vi "nanocal -- nuclear schottky fit V3.vi"() -> ()   [LabVIEW 2020] (continued)
  T4 = typedef "nameformattingitem.ctl" = enum16{"name", "nameL", "units", "prec"}
  T5 = typedef "nanocal-goodness-weighting-strategy.ctl" = enum16{"dω", "dω √(|dz/dω|)", "dω |dz/dω|", "phase", "andreas", "sum"}
  T6 = typedef "3-lorentzian-heat-response action.ctl" = enum16{"calc R", "create string", "calc m1m2m3", "dζ", "dT1", "dτS", "dτN", "dτC", "d-all", "dκ0", "T(K)", "m1", "m2", "m3", "parse string", "θ (deg)", "B (T)", "onlygrads", "newton", "create emty string"}
  T7 = enum32{"main", "parameters", "ignore", "save scan"}
  T8 = typedef "cursor winow.ctl" = cluster{"left":dbl, "right ":dbl, "center":dbl, "window":dbl, "cursors":i32[], "relative":i32, "absolute":i32, "fixed vertical offset":dbl, "vertical offset":dbl, "skew":dbl, "default window frac":dbl, "kind":enum16{"symmetric", "skewed", "fancy"}, "skew.left":dbl, "skew.right":dbl, "Plot ref":refnum<vi>, "wing order":enum16{"forw", "back"}}
  T9 = typedef "show-win- control.ctl" = cluster{"cen (Hz)":dbl, "win (Hz)":dbl, "left (Hz)":dbl, "right (Hz)":dbl}
  T10 = typedef "NI_Gmath.lvlib/stopping criteria.ctl" = cluster{"function tolerance":dbl, "parameter tolerance":dbl, "max iterations":i32, "max function calls":i32, "gradient tolerance":dbl, "max time (sec)":dbl}
  T11 = typedef "filename-pattern.ctl" = cluster{"prefix":string, "group":string}
  T12 = typedef "cursor action.ctl" = enum16{"range", "read", "write", "check", "zoom out", "smart zoom out", "zoom to aspect ratio 1", "zoom to win", "zoom out 20%", "zoom in 20%", "-empty", "smart zoom out&aspect", "move range left 20%", "move range right 20%", "move range up 20%", "move range down 20%", "zoom to X win", "zoom to Y win", "zoom out X", "zoom out Y", "zoom in X", "zoom in Y", "check plot scale", "set color", "set Xlabel", "set Ylabel"}
  T13 = typedef "cursor window action.ctl" = enum16{"balance", "h. offset change", "cursor moves", "change center", "change window", "init", "check", "reset", "set y to middle", "idle", "-write all Y", "-write left.X", "-write center.X", "-write right.X", "-write all X", "-change center", "-change window", "-change skew", "-read cursor 2", "-read cursor 1", "-read cursor 0", "-read all cursors", "-reset", "-read plot scale", "-set y to middle", "-Q: center.Y is visible", "-Q: window is visible", "-parse center.Y", "-right left from center", "-left move", "-right move", "-set center.Y", "-empty", "-set cursors to default", "-check", "-write center.Y", "-copy cursor 1", "-copy cursor 0", "-copy cursor 2", "move right", "move left", "shrink", "broaden", "skew up", "skew down", "-write plot scale", "zoom X", "change cen&win", "zoom to all data", "color--red", "color--green", "color--yellow", "read", "zoom out", "zoom in", "slide right", "slide left", "set range aspect ratio to 1"}
  T14 = typedef "mathematica string map action.ctl" = enum16{"create string", "calc m1m2m3", "parse string"}
  T15 = typedef "publisher action.ctl" = enum16{"set", "get", "init", "check"}
  T16 = typedef "cursor sate.ctl" = enum16{"normal", "alert", "fuzzy", "interesting", "boring", "colored"}
  T17 = typedef "3-lorentzian-parameters -- action.ctl" = enum16{"to array", "to parameters"}
  T18 = typedef "NI_Gmath.lvlib/objective function data.ctl" = variant
  T19 = typedef "filename-action.ctl" = enum16{"rewrite", "parse", "force pattern", "uniquenum", "get T", "get B", "get ind", "get deg", "get name", "get folder", "get extension", "get basename", "get side", "get change"}
  T20 = typedef "LVMapReplaceAction.ctl" = enum32{"Modify Entry only if found", "Add or Modify Entry", "Delete Entry"}
  T21 = typedef "file -- read-write control.ctl" = enum16{"read", "write all", "append one line"}
  T22 = typedef "array -- freq-voltage transformations action.ctl" = enum16{"as is", "add -ω", "sort ω", "2 x ω", "R-phase(deg) to Re-Im", "select ω>0"}
  T23 = typedef "nanocal_raw_file_manage_action_V1.ctl" = enum16{"read S side", "read R side", "read meta", "read_names"}
  T24 = typedef "KM_file -- read-write control.ctl" = enum16{"read", "write all", "append one line"}
  T25 = typedef "array action.ctl" = enum16{"generate range", "generate log range"}
  T26 = typedef "LVRangeTypeDef.ctl" = cluster{"Minimum":dbl, "Maximum":dbl, "Increment":dbl, "Minor Increment":dbl, "Start":dbl}
  T27 = typedef "2Dwindow.ctl" = cluster{"window y":dbl, "center x":dbl, "center y":dbl, "window x":dbl}
  T28 = typedef "eventvkey.ctl" = enum16{"ASCII", "Enter", "Return", "Shift", "Ctrl", "Alt", "Cmd", "Opt", "Caps", "NumLock", "Clear", "Break", "Up", "Down", "Left", "Right", "Insert", "Delete", "Home", "End", "PageUp", "PageDown", "Escape", "Help", "Pause", "ScrollLock", "F1", "F2", "F3", "F4", "F5", "F6", "F7", "F8", "F9", "F10", "F11", "F12", "F13", "F14", "F15", "F16", "F17", "F18", "F19", "F20", "F21", "F22", "F23", "F24", "Play", "VolumeUp", "VolumeDown", "Mute", "Two Byte Char"}
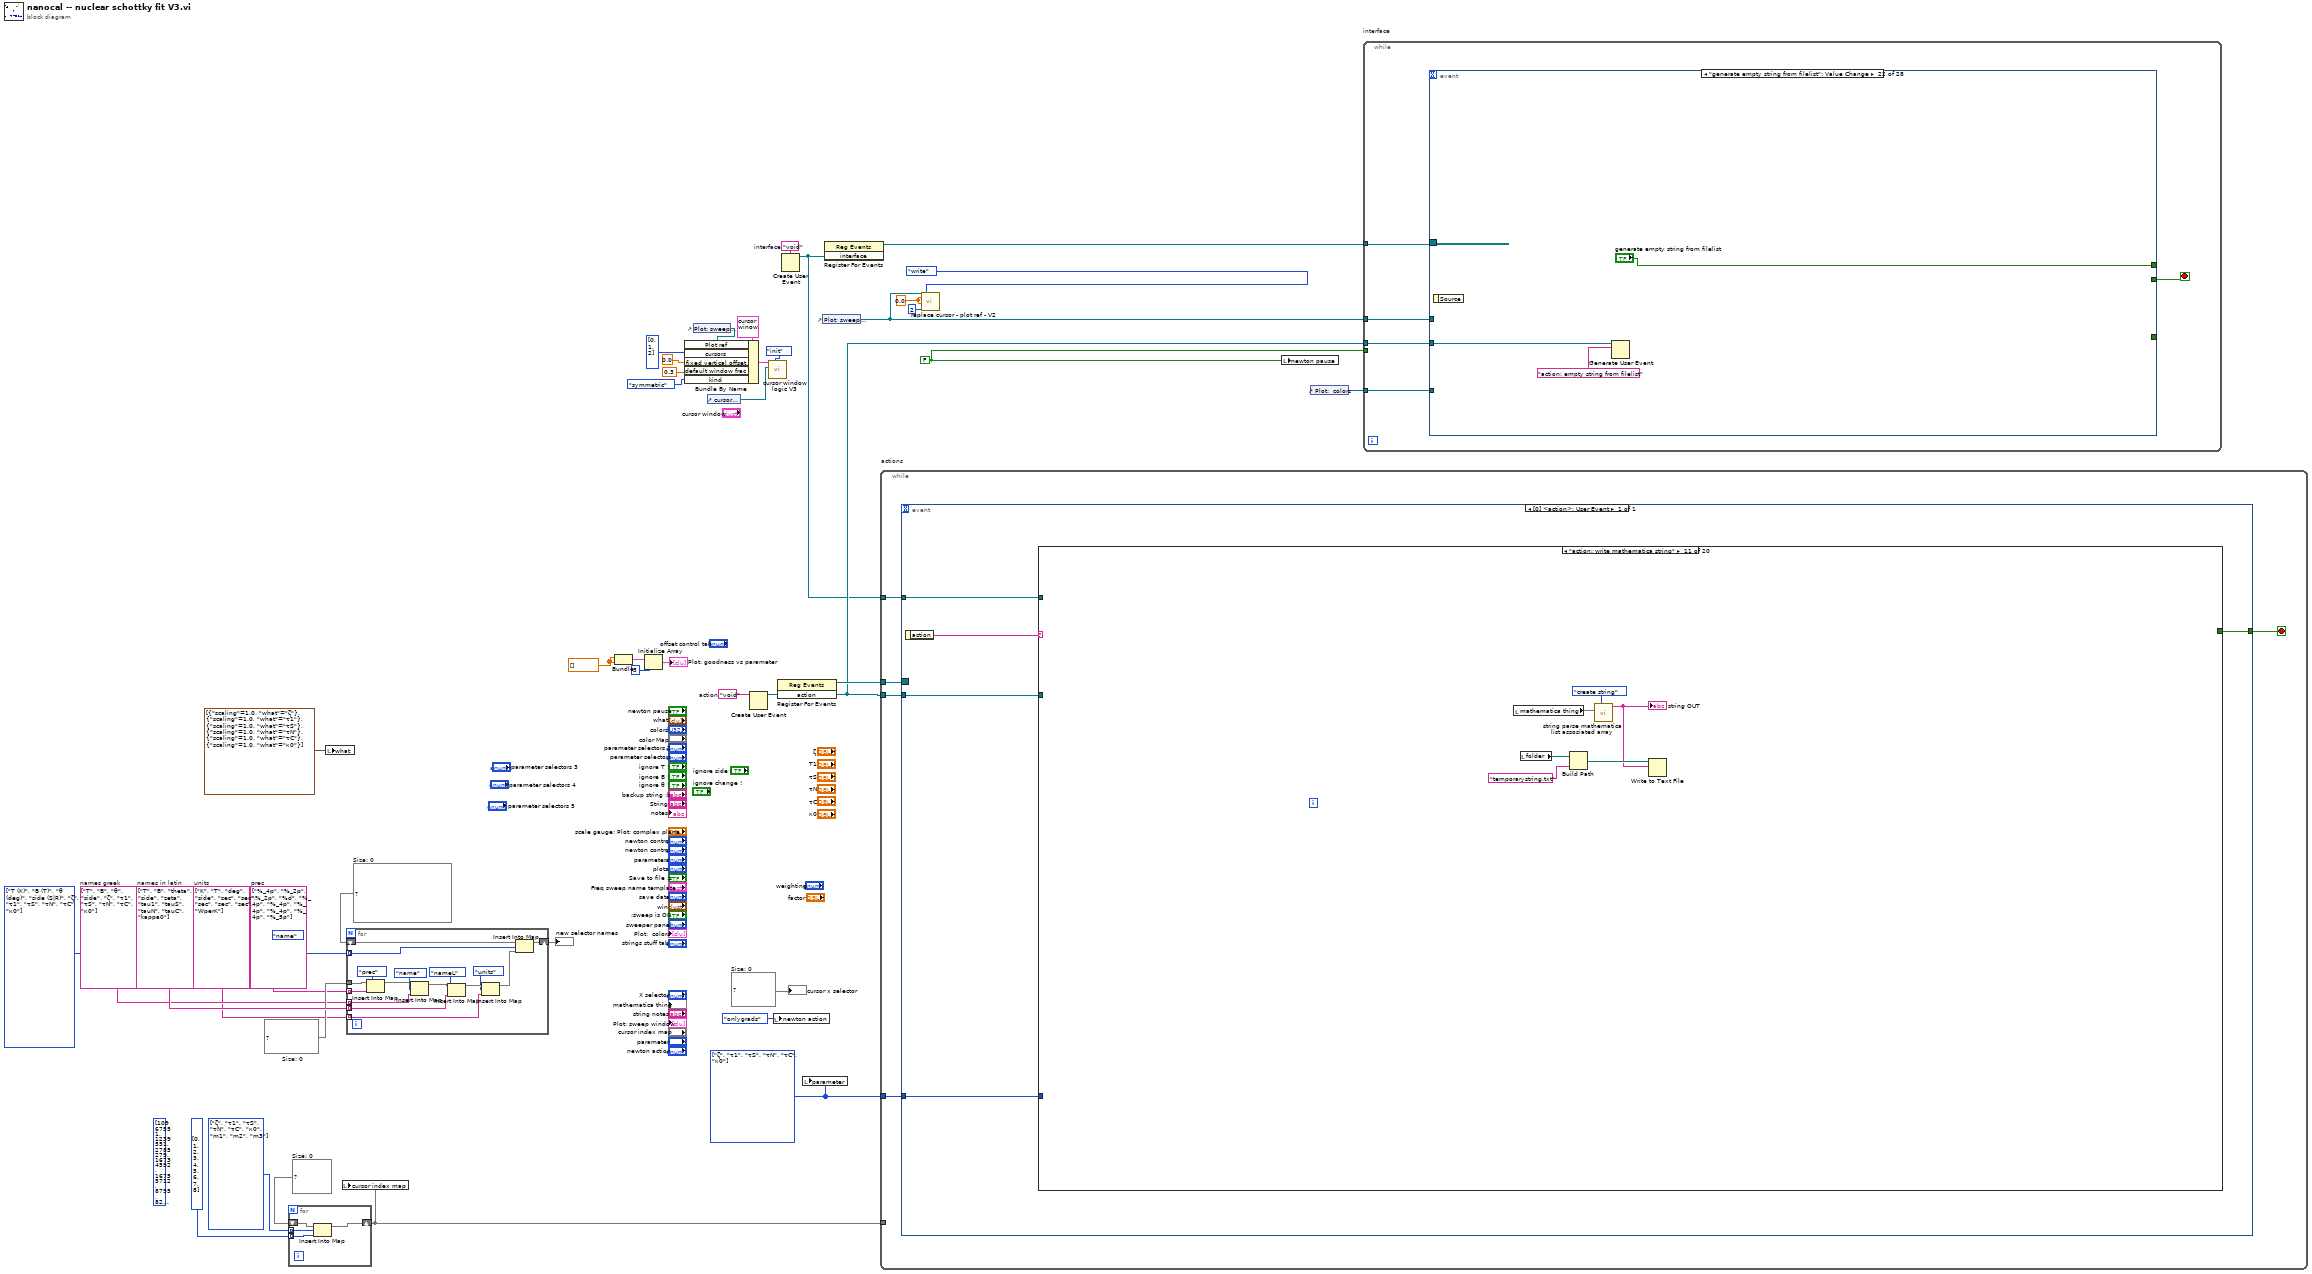
[diagram p0: block diagram]
diagram:
  w1 = string[] ["%_4p", "%_2p", "%_2p", "%d", "%_4p", "%_4p", "%_4p", "%_4p", "%_4p", "%_5p"]  # prec
  w5 = map{T4, string} {}  # Size: 0
  (unwired) nameformattingitem."name" ("name formatting item")
  w3 = string[] ["K", "T", "deg", "side", "sec", "sec", "sec", "sec", "sec", "WperK"]  # units
  w6 = string[] ["T", "B", "theta", "side", "zeta", "tau1", "tauS", "tauN", "tauC", "kappa0"]  # names in latin
  w4 = string[] ["T", "B", "θ", "side", "ζ", "τ1", "τS", "τN", "τC", "κ0"]  # names greek
  w8 = map{T1, map{T4, string}} {}  # Size: 0
  w7 = T1[] [enum."T (K)", enum."B (T)", enum."θ (deg)", enum."side (S|R)", enum."ζ", enum."τ1", enum."τS", enum."τN", enum."τC", enum."κ0"] items=["ζ", "τ1", "τS", "τN", "τC", "κ0", "m1", "m2", "m3", "T (K)", "B (T)", "θ (deg)", "side (S|R)", "change (B|T)"]
  w14 = dbl[] []
  (unwired) u32[] [10967551, 1239551, 2785279, 16734592, 16755712, 8795, 8285330, 9272482, 9204890]
  w10 = T1[] [enum."ζ", enum."τ1", enum."τS", enum."τN", enum."τC", enum."κ0"] items=["ζ", "τ1", "τS", "τN", "τC", "κ0", "m1", "m2", "m3", "T (K)", "B (T)", "θ (deg)", "side (S|R)", "change (B|T)"]
  w20 = map{T1, i32} {}  # Size: 0
  w15 = T1[] [enum."ζ", enum."τ1", enum."τS", enum."τN", enum."τC", enum."κ0", enum."m1", enum."m2", enum."m3"] items=["ζ", "τ1", "τS", "τN", "τC", "κ0", "m1", "m2", "m3", "T (K)", "B (T)", "θ (deg)", "side (S|R)", "change (B|T)"]
  w21 = FALSE ("newton pause")
  w23 = map{T1, dbl} {}  # Size: 0
  w24 = 0.0 ("new X")
  w38 = "void"  # interface
  w40 = "void"  # action
  n1 = for {
    shift-right: [w44] -> w18
    shift-left: w20 -> [w45]
    tunnel: w15 -> [w43] mode=indexing
    tunnel: i32[] [0, 1, 2, 3, 4, 5, 6, 7, 8] -> [w42] mode=indexing
    n2 = Insert Into Map(map in=w45, key=w43, value=w42) -> (map out=w44:map{T1, i32})  [unwired: 2 out]
  }
  n3 = local write "what"(cluster{"scaling":dbl, "what":T1}[] [{"scaling"=1.0, "what"=enum."ζ"}, {"scaling"=1.0, "what"=enum."τ1"}, {"scaling"=1.0, "what"=enum."τS"}, {"scaling"=1.0, "what"=enum."τN"}, {"scaling"=1.0, "what"=enum."τC"}, {"scaling"=1.0, "what"=enum."κ0"}]) -> ()
  n4 = local write "cursor index map"(w18) -> ()
  n5 = for {
    shift-right: [w60] -> w2
    shift-left: w8 -> [w61]
    tunnel: w6 -> [w51] mode=indexing
    tunnel: w7 -> [w59] mode=indexing
    tunnel: w5 -> [w49]
    tunnel: w4 -> [w50] mode=indexing
    tunnel: w3 -> [w52] mode=indexing
    tunnel: w1 -> [w48] mode=indexing
    n6 = Insert Into Map(map in=w49, key=nameformattingitem."prec", value=w48) -> (map out=w47:map{T4, string})  [unwired: 2 out]
    n7 = Insert Into Map(map in=w47, key=nameformattingitem."name", value=w50) -> (map out=w58:map{T4, string})  [unwired: 2 out]
    n8 = Insert Into Map(map in=w58, key=nameformattingitem."nameL" ("name formatting item"), value=w51) -> (map out=w57:map{T4, string})  [unwired: 2 out]
    n9 = Insert Into Map(map in=w57, key=nameformattingitem."units" ("name formatting item"), value=w52) -> (map out=w56:map{T4, string})  [unwired: 2 out]
    n10 = Insert Into Map(map in=w61, key=w59, value=w56) -> (map out=w60:map{T1, map{T4, string}})  [unwired: 2 out]
  }
  "new selector names" <- w2
  n11 = Bundle(w14, w14) -> (w13:cluster{dbl[], dbl[]})  [unwired: 1 in]
  n12 = Initialize Array(w13, 5 ("dimension size")) -> (→"Plot: goodness vs parameter":cluster{dbl[], dbl[]}[])
  n13 = control-ref of="Plot: sweep window"() -> (w30:refnum<vi>)
  n14 = Bundle By Name(cluster=T8 {"left"=0.0, "right "=0.0, "center"=0.0, "window"=0.0, "cursors"=[], "relative"=0, "absolute"=0, "fixed vertical offset"=0.0, "vertical offset"=0.0, "skew"=0.0, "default window frac"=0.0, "kind"=enum."symmetric", "skew.left"=0.0, "skew.right"=0.0, "Plot ref"=refnum, "wing order"=enum."forw"} ("cursor bracket: All, data window"), "Plot ref"=w30, "cursors"=i32[] [0, 1, 2], "fixed vertical offset"=0.0, "default window frac"=0.3 ("fixed vertical offset"), "kind"=enum16{"symmetric", "skewed", "fancy"}."symmetric") -> (w33:T8)
  n15 = control-ref of="cursor window"() -> (w29:refnum<vi>)
  n16 = Create User Event(user event datatype=w40) -> (user event=w28:refnum<user-event>)  [unwired: 1 in, 1 out]
  n17 = call "cursor window logic V3.vi"("cursor window action"=cursor_window_action."init", "cursor window in"=w29, "cursor window init"=w33) -> ()  [unwired: 7 in, 2 out]
  n18 = local write "newton action"(3-lorentzian-heat-response_action."onlygrads" ("newton action")) -> ()
  n19 = register-events(w28) -> (reference out=w41:refnum<event-registration>)  [unwired: 2 in, 1 out]
  n20 = Create User Event(user event datatype=w38) -> (user event=w16:refnum<user-event>)  [unwired: 1 in, 1 out]
  n21 = local write "parameter"(w10) -> ()
  n22 = control-ref of="Plot: sweep window"() -> (w25:refnum<vi>)
  n23 = register-events(w16) -> (reference out=w39:refnum<event-registration>)  [unwired: 2 in, 1 out]
  n24 = while "actions" {
    tunnel: w41 -> [w66]
    tunnel: w28 -> [w65]
    tunnel: w18 -> [_]
    tunnel: w16 -> [w63]
    tunnel: w10 -> [w62]
    stop <- w64 stop-if-true
    n25 = event shown="[0] <action>: User Event" {
      selector: w66 -> [_]
      dyn-events: _ -> [_]
      timeout: _ -> [_]
      tunnel: w65 -> [w70]
      tunnel: [w69] -> w64
      tunnel: w63 -> [w68]
      tunnel: w62 -> [w67]
      event User Event {
        n26 = event-data() -> ("action"=w71:string)  [unwired: 1 in]
        n27 = case shown="\"action: write mathematica string\"" w71 {
          tunnel: w70 -> [w72 _ _ w324 w431 w449 w462 _ w573 _ _ _ w807 _ w885 w924 _ w977 _ _]
          tunnel: [_ _ _ _ _ _ _ _ _ _ _ _ _ _ _ _ TRUE _ _ _] -> w69
          tunnel: w68 -> [_ _ _ w323 _ _ _ _ _ _ _ _ _ _ _ _ _ _ _ _]
          tunnel: w67 -> [w74 w151 w207 _ _ _ _ _ _ _ _ w724 _ _ _ _ _ _ _ _]
          frame "action: new sweep" {
            (unwired) 3-lorentzian-heat-response_action."onlygrads" ("action")
            w80 = T1[] [enum."m1", enum."m2", enum."m3"] items=["ζ", "τ1", "τS", "τN", "τC", "κ0", "m1", "m2", "m3", "T (K)", "B (T)", "θ (deg)", "side (S|R)", "change (B|T)"]
            w86 = T1[] [enum."T (K)", enum."B (T)", enum."θ (deg)"] items=["ζ", "τ1", "τS", "τN", "τC", "κ0", "m1", "m2", "m3", "T (K)", "B (T)", "θ (deg)", "side (S|R)", "change (B|T)"]
            w123 = 6.283185307179586
            n28 = Generate User Event(user event=w72, event data cluster="action: reset colors" ("event data")) -> ()  [unwired: 2 in, 2 out]
            n29 = local read "T1"() -> (w109:dbl)
            n30 = call "nanocal -- publish -- freq scan V2.vi"("publisher action"=publisher_action."get") -> ("dz/dω out (V)"=w124:cdb[], "z out (V)"=w119:cdb[], "ω out (Hz)"=w126:dbl[])  [unwired: 8 in]
            n31 = local read "τS"() -> (w108:dbl)
            n32 = local read "τN"() -> (w107:dbl)
            n33 = local read "τC"() -> (w106:dbl)
            n34 = local read "κ0"() -> (w105:dbl)
            n35 = local read "ζ"() -> (w110:dbl)
            n36 = Divide(x=w124, y=w123) -> (x/y=w121:cdb[])
            n37 = Multiply(x=w126, y=w123) -> (x*y=w118:dbl[])
            n38 = Build Array (concatenate)(w74, w80) -> (w79:T1[])
            n39 = Build Array(w110, w109, w108, w107, w106, w105) -> (w92:dbl[])
            n40 = local read "newton action"() -> (w75:T6)
            n41 = for {
              shift-right: [w137] -> w78
              shift-left: map{T1, dbl} {} ("Map IN") -> [w138]
              tunnel: w79 -> [w135] mode=indexing
              tunnel: w92 -> [w136] mode=indexing
              tunnel: [w135] -> w81 mode=indexing
              n42 = Insert Into Map(map in=w138, key=w135, value=w136) -> (map out=w137:map{T1, dbl})  [unwired: 2 out]
            }
            n43 = local read "weighting"() -> (w120:T5)
            n44 = call "nanocal -- nuclear schottky goodness V5.vi"("action"=w75, "parameters IN"=w78, "weighting strategy"=w120, "dz/dω IN (V)"=w121, "Voltage IN (V)"=w119, "ω (rad/sec)"=w118) -> ("R norm"=w117:dbl, "G"=w116:dbl, "R(ω) out"=w115:cdb[], "dG / d log α   OUT"=w77:map{T1, dbl})  [unwired: 2 in]
            n45 = for {
              tunnel: w74 -> [w129] mode=indexing
              shift-right: [w130] -> _
              shift-left: w77 -> [w130]
              tunnel: [w128] -> w76 mode=indexing
              n46 = Look In Map(map=w130, key=w129) -> (value=w128:dbl)  [unwired: 1 in, 1 out]
            }
            "logarithmic derivatives" <- w76
            n47 = Divide(x=w116, y=w117) -> (x/y=→"goodness":dbl)
            n48 = local read "θ (deg)"() -> (w88:dbl)
            n49 = local read "B (T)"() -> (w89:dbl)
            n50 = local read "T (K)"() -> (w90:dbl)
            n51 = call "3-lorentzian-heat-response -- V4.vi"("action"=3-lorentzian-heat-response_action."calc m1m2m3", "Map IN"=w78) -> ("Map OUT"=w87:map{T1, dbl})  [unwired: 7 in, 2 out]
            n52 = Build Array(w90, w89, w88) -> (w85:dbl[])
            n53 = local read "cursor x selector"() -> (w114:map{T1, dbl})
            n54 = local read "X selector"() -> (w113:T1)
            n55 = local read "cursor index map"() -> (w94:map{T1, i32})
            n56 = for {
              shift-right: [w133] -> w84
              shift-left: w87 -> [w134]
              tunnel: w86 -> [w132] mode=indexing
              tunnel: w85 -> [w131] mode=indexing
              n57 = Insert Into Map(map in=w134, key=w132, value=w131) -> (map out=w133:map{T1, dbl})  [unwired: 2 out]
            }
            n58 = local read "T (K)"() -> (w112:dbl)
            n59 = control-ref of="Plot:  colors"() -> (w125:refnum<vi>)
            n60 = control-ref of="Plot: sweep window"() -> (w104:refnum<vi>)
            n61 = Complex To Re/Im(x + iy=w119) -> (x=w103:dbl[], y=w102:dbl[])
            n62 = Look In Map(map=w114, key=w113, default value=w112) -> (value=w111:dbl)  [unwired: 1 out]
            n63 = call "replace plot - plot ref - V2.vi"("Plot ref in"=w104, "Array X IN"=w103, "Array Y IN"=w102, "plot index"=enum16{"data R(ω)", "fit R(ω)"}."data R(ω)" ("Plost: sweep window"), "cursor action"=cursor_action."write") -> ("Plot ref out"=w101:refnum<vi>)  [unwired: 11 in, 3 out]
            n64 = for {
              tunnel: w111 -> [w146]
              tunnel: w125 -> [w145]
              tunnel: w81 -> [w141] mode=indexing
              tunnel: w94 -> [w143]
              shift-right: [w140] -> _
              shift-left: w87 -> [w140]
              n65 = Look In Map(map=w140, key=w141) -> (value=w139:dbl)  [unwired: 1 in, 1 out]
              n66 = Look In Map(map=w143, key=w141) -> (value=w142:i32)  [unwired: 1 in, 1 out]
              n67 = call "replace cursor - plot ref - V2.vi"("Plot ref in"=w145, "new X"=w146, "new  Y"=w139, "cursor index"=w142, "cursor action"=cursor_action."write") -> ()  [unwired: 11 in, 4 out]
            }
            n68 = call "string parse mathematica assosiated array.vi"("derivative"=mathematica_string_map_action."create string", "Map IN"=w84) -> ("String OUT"=w82:string)  [unwired: 8 in, 1 out]
            n69 = Complex To Re/Im(x + iy=w115) -> (x=w99:dbl[], y=w98:dbl[])
            n70 = local write "String"(w82) -> ()
            n71 = call "replace plot - plot ref - V2.vi"("Plot ref in"=w101, "Array X IN"=w99, "Array Y IN"=w98, "plot index"=enum16{"data R(ω)", "fit R(ω)"}."fit R(ω)" ("Plost: sweep window"), "cursor action"=cursor_action."write") -> ()  [unwired: 11 in, 4 out]
          }
          frame "action: replot circles" {
            w179 = 6.283185307179586
            n72 = call "nanocal -- publish -- freq scan V2.vi"("publisher action"=publisher_action."get") -> ("dz/dω out (V)"=w180:cdb[], "z out (V)"=w176:cdb[], "ω out (Hz)"=w181:dbl[])  [unwired: 8 in]
            n73 = local read "T1"() -> (w170:dbl)
            n74 = local read "τS"() -> (w169:dbl)
            n75 = local read "κ0"() -> (w166:dbl)
            n76 = local read "τN"() -> (w168:dbl)
            n77 = local read "τC"() -> (w167:dbl)
            n78 = local read "ζ"() -> (w171:dbl)
            n79 = Divide(x=w180, y=w179) -> (x/y=w178:cdb[])
            n80 = Multiply(x=w181, y=w179) -> (x*y=w175:dbl[])
            n81 = Build Array(w171, w170, w169, w168, w167, w166) -> (w152:dbl[])
            n82 = for {
              shift-right: [w188] -> w150
              shift-left: map{T1, dbl} {} ("Map IN") -> [w189]
              tunnel: w151 -> [w187] mode=indexing
              tunnel: [w186] -> _ mode=indexing
              tunnel: [w187] -> w148 mode=indexing
              tunnel: w152 -> [w186] mode=indexing
              n83 = Insert Into Map(map in=w189, key=w187, value=w186) -> (map out=w188:map{T1, dbl})  [unwired: 2 out]
            }
            n84 = local read "weighting"() -> (w177:T5)
            n85 = call "nanocal -- nuclear schottky goodness V5.vi"("action"=3-lorentzian-heat-response_action."onlygrads", "parameters IN"=w150, "weighting strategy"=w177, "dz/dω IN (V)"=w178, "Voltage IN (V)"=w176, "ω (rad/sec)"=w175) -> ("R norm"=w174:dbl, "G"=w173:dbl, "R(ω) out"=w172:cdb[], "dG / d log α   OUT"=w149:map{T1, dbl})  [unwired: 2 in]
            n86 = control-ref of="Plot: sweep window"() -> (w162:refnum<vi>)
            n87 = Divide(x=w173, y=w174) -> (x/y=w165:dbl)
            n88 = for {
              tunnel: w148 -> [w184] mode=indexing
              shift-right: [w185] -> _
              shift-left: w149 -> [w185]
              tunnel: [w183] -> w147 mode=indexing
              n89 = Look In Map(map=w185, key=w184) -> (value=w183:dbl)  [unwired: 1 in, 1 out]
            }
            n90 = Complex To Re/Im(x + iy=w176) -> (x=w160:dbl[], y=w159:dbl[])
            n91 = local write "goodness"(w165) -> ()
            n92 = call "replace plot - plot ref - V2.vi"("Plot ref in"=w162, "Array X IN"=w160, "Array Y IN"=w159, "plot index"=enum16{"data R(ω)", "fit R(ω)"}."data R(ω)" ("Plost: sweep window"), "cursor action"=cursor_action."write") -> ("Plot ref out"=w161:refnum<vi>)  [unwired: 11 in, 3 out]
            n93 = Complex To Re/Im(x + iy=w172) -> (x=w158:dbl[], y=w157:dbl[])
            n94 = local write "logarithmic derivatives"(w147) -> ()
            n95 = call "replace plot - plot ref - V2.vi"("Plot ref in"=w161, "Array X IN"=w158, "Array Y IN"=w157, "plot index"=enum16{"data R(ω)", "fit R(ω)"}."fit R(ω)" ("Plost: sweep window"), "cursor action"=cursor_action."write") -> ()  [unwired: 11 in, 4 out]
          }
          frame "action: plot landscape" {
            w199 = array_action."generate log range" ("action")
            w221 = 6.283185307179586
            n96 = property on="range one" class="Slide (strict)"() -> ("Scale.Range"=w211:T26)  [unwired: 2 in, 2 out]
            n97 = property on="range two" class="Slide (strict)"() -> ("Scale.Range"=w210:T26)  [unwired: 2 in, 2 out]
            n98 = Unbundle By Name(w211) -> ("Maximum"=w202:dbl, "Minimum"=w201:dbl)
            n99 = Unbundle By Name(w210) -> ("Maximum"=w204:dbl, "Minimum"=w203:dbl)
            n100 = local read "ζ"() -> (w217:dbl)
            n101 = local read "T1"() -> (w216:dbl)
            n102 = local read "τS"() -> (w215:dbl)
            n103 = local read "τN"() -> (w214:dbl)
            n104 = local read "τC"() -> (w213:dbl)
            n105 = local read "κ0"() -> (w212:dbl)
            n106 = call "nanocal -- publish -- freq scan V2.vi"("publisher action"=publisher_action."get") -> ("dz/dω out (V)"=w222:cdb[], "z out (V)"=w219:cdb[], "ω out (Hz)"=w223:dbl[])  [unwired: 8 in]
            n107 = local read "cursor index map"() -> (w193:map{T1, i32})
            n108 = Build Array(w217, w216, w215, w214, w213, w212) -> (w198:dbl[])
            n109 = call "array -- generate range -- V5.vi"("action"=w199, "ω points"="# points", "ω from"=w201, "ω to"=w202) -> ("ω out"=w200:dbl[])  [unwired: 7 in]
            n110 = call "array -- generate range -- V5.vi"("action"=w199, "ω points"="# points", "ω from"=w203, "ω to"=w204) -> ("ω out"=w205:dbl[])  [unwired: 7 in]
            n111 = local read "color Map"() -> (w194:map{T1, u32})
            n112 = Divide(x=w222, y=w221) -> (x/y=w220:cdb[])
            n113 = Multiply(x=w223, y=w221) -> (x*y=w218:dbl[])
            n114 = for {
              shift-right: [w314] -> w206
              shift-left: map{T1, dbl} {} ("Map IN") -> [w315]
              tunnel: w207 -> [w313] mode=indexing
              tunnel: w198 -> [w312] mode=indexing
              n115 = Insert Into Map(map in=w315, key=w313, value=w312) -> (map out=w314:map{T1, dbl})  [unwired: 2 out]
            }
            n116 = Look In Map(map=w194, key="one") -> (value=w195:u32)  [unwired: 1 in, 1 out]
            n117 = Look In Map(map=w194, key="two") -> (value=w196:u32)  [unwired: 1 in, 1 out]
            n118 = property on="range one" class="Slide (strict)"("Fill Color"=w195) -> ()  [unwired: 2 in, 2 out]
            n119 = property on="range two" class="Slide (strict)"("Fill Color"=w196) -> ()  [unwired: 2 in, 2 out]
            n120 = Build Array("one", "two") -> (w192:T1[])
            n121 = case shown="\"1d plots\", Default" "what" {
              tunnel: w220 -> [w233 w276]
              tunnel: w219 -> [w232 w275]
              tunnel: w218 -> [w231 w274]
              tunnel: w206 -> [w230 w273]
              tunnel: "one" -> [_ w272]
              tunnel: w205 -> [_ w271]
              tunnel: w200 -> [w229 w270]
              tunnel: "two" -> [_ w269]
              tunnel: w194 -> [w228 _]
              tunnel: w193 -> [w227 _]
              tunnel: w192 -> [w225 _]
              frame "1d plots", Default {
                n122 = control-ref of="Plot: goodness vs parameter"() -> (w226:refnum<vi>)
                n123 = for {
                  tunnel: w233 -> [w252]
                  tunnel: w232 -> [w251]
                  tunnel: w231 -> [w250]
                  tunnel: w230 -> [w237]
                  tunnel: w229 -> [w246]
                  tunnel: w225 -> [w236] mode=indexing
                  tunnel: w228 -> [w243]
                  tunnel: w227 -> [w242]
                  tunnel: w226 -> [w234]
